vi "VisionPose.vi"(5 "Odometry Delta Y (in) [t0]":dbl, 6 "Vision Trust Threshold (in)":dbl, 7 "Odometry Delta X (in) [t0]":dbl, 10 "AprilTag Data [t-?]":dbl[](array[numeric]), 11 "Vision Target Valid [t-?]":bool) -> (1 "Vision Y (in) [t-?]":dbl, 2 "Vision X (in) [t-?]":dbl, 3 "Vision Valid [t-?]":bool)   [LabVIEW 2020]
doc: "Calculates the robot pose using the AprilTag data from the LimeLight camera. Also performs additional validation checks to determine if the vision data should be trusted."
uses:
  d330619a-1645-40d1-9d50-519401bd8c1e.vi
  4285d199-8f61-4066-b628-7d31460b52c1.vi
  GlobalPoseAndTargeting.vi
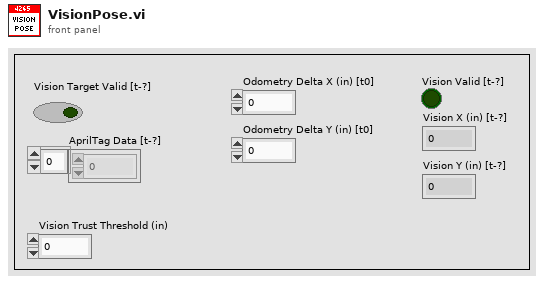
[diagram p1: front panel]
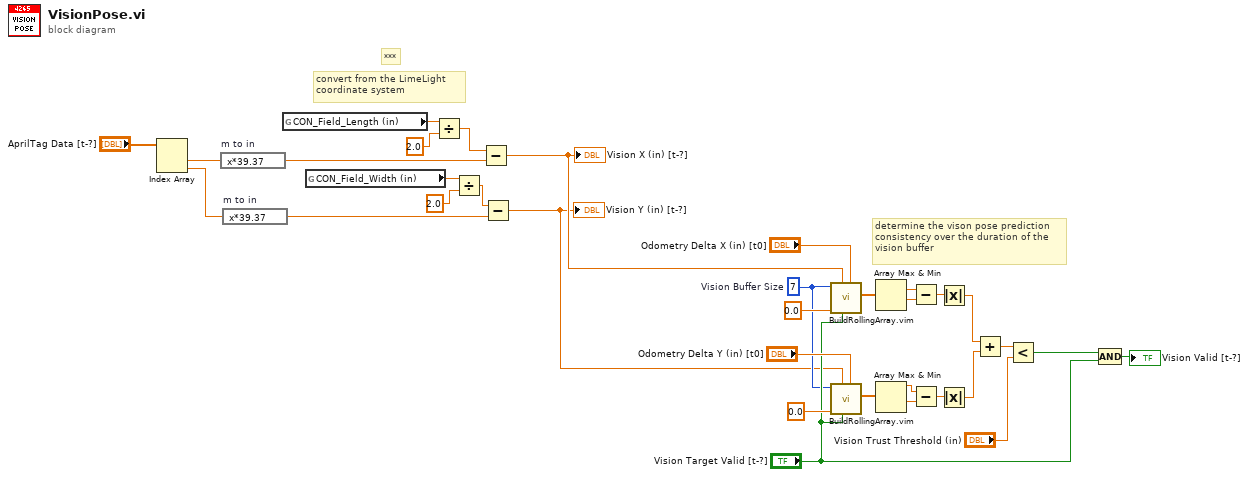
[diagram p0: block diagram]
diagram:
  w14 = 7  # Vision Buffer Size
  # "***"
  # "convert from the LimeLight\ncoordinate system"
  # "determine the vison pose prediction\nconsistency over the duration of the\nvision buffer"
  n1 = Index Array(array="AprilTag Data [t-?]") -> (element #1=w4:dbl, element #2=w2:dbl)  [unwired: 2 in]
  n2 = expression code="x*39.37" "m to in"(w4) -> (w3:dbl)
  n3 = expression code="x*39.37" "m to in"(w2) -> (w1:dbl)
  n4 = global read "GlobalPoseAndTargeting.vi" "CON_Field_Length (in)"() -> (w10:dbl)
  n5 = global read "GlobalPoseAndTargeting.vi" "CON_Field_Width (in)"() -> (w7:dbl)
  n6 = Divide(x=w10, y=2.0) -> (x/y=w8:dbl)
  n7 = Divide(x=w7, y=2.0) -> (x/y=w5:dbl)
  n8 = Subtract(x=w8, y=w3) -> (x-y=w12:dbl)
  "Vision X (in) [t-?]" <- w12
  n9 = Subtract(x=w5, y=w1) -> (x-y=w11:dbl)
  "Vision Y (in) [t-?]" <- w11
  n10 = call "BuildRollingArray.vim"("Global Additive Update"="Odometry Delta X (in) [t0]", "Update?"="Vision Target Valid [t-?]", "New Value"=w12, "Initial Value"=0.0, "Number of Elements"=w14) -> ("Current Array"=w27:dbl[])  [unwired: 6 in]
  n11 = call "BuildRollingArray.vim"("Global Additive Update"="Odometry Delta Y (in) [t0]", "Update?"="Vision Target Valid [t-?]", "New Value"=w11, "Initial Value"=0.0, "Number of Elements"=w14) -> ("Current Array"=w22:dbl[])  [unwired: 6 in]
  n12 = Array Max & Min(array=w27) -> (max value=w26:dbl, min value=w25:dbl)  [unwired: 2 out]
  n13 = Array Max & Min(array=w22) -> (max value=w21:dbl, min value=w23:dbl)  [unwired: 2 out]
  n14 = Subtract(x=w26, y=w25) -> (x-y=w29:dbl)
  n15 = Subtract(x=w21, y=w23) -> (x-y=w24:dbl)
  n16 = Absolute Value(x=w29) -> (abs(x)=w28:dbl)
  n17 = Absolute Value(x=w24) -> (abs(x)=w20:dbl)
  n18 = Add(x=w28, y=w20) -> (x+y=w30:dbl)
  n19 = Less?(x=w30, y="Vision Trust Threshold (in)") -> (x < y?=w19:bool)
  n20 = Compound Arithmetic op=AND(w19, "Vision Target Valid [t-?]") -> (→"Vision Valid [t-?]":bool)
